vi "InitDone.vi"(8 "error in (no error)":errorcluster, 10 "Variant":variant, 11 "SpectrometerUI in":refnum<class "SpectrometerUI.lvclass">) -> (0 "error out":errorcluster, 3 "SpectrometerUI out":refnum<class "SpectrometerUI.lvclass">)   [LabVIEW 2023, in "SpectrometerUI.lvlib" / "SpectrometerUI.lvclass"]
uses:
  SpectrometerUI.lvclass
  SpectrometerUI.lvclass/SpectrometerUI.ctl
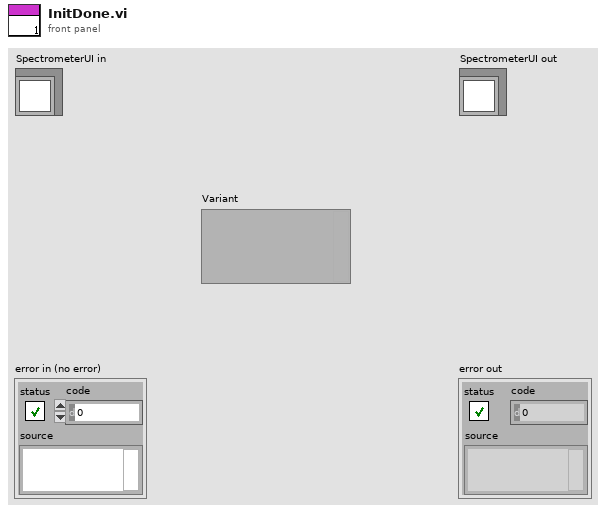
[diagram p1: front panel]
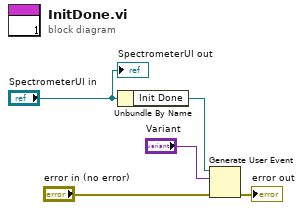
[diagram p0: block diagram]
diagram:
  n1 = Unbundle By Name("SpectrometerUI in") -> ("Init Done"=w4:refnum<user-event>)
  n2 = Generate User Event(user event=w4, event data cluster="Variant", error in="error in (no error)") -> (error out=→"error out":errorcluster)  [unwired: 1 in, 1 out]
  "SpectrometerUI out" <- "SpectrometerUI in"
